vi "set poisition.vi"(4 "Mode":u16(ring) items=["Move to position", "Move to limit", "Redefine current position"], 5 "Instrument":T1={"325 Resource "="GPIB0::13::INSTR", "Input (0:A) 325"=0, "Heater Output (1:1) 325"=1, "340 Resource"="GPIB0::14::INSTR", "Input (0:A) 340"=0, "Loop (0: 1)"=0, "Input (0:B) 340"=1, "Loop (1: 1)"=0, "340 Status"=refnum, "Instrument Type"=enum."PPMS-Rotate", "quantum design"=refnum, "semaphore 325"=refnum, "TCP master instance"=refnum, "M24C Resource"="GPIB0::24::INSTR", "4G supply"="GPIB0::24::INSTR", "Temp Status 24C"=refnum, "Temp"=refnum, "9T信号"=refnum, "limit"={"Field limit"=0.0, "Field rate limit"=0.0, "Temp limit"=0.0, "Temp low limit"=0.0, "Temp rate limit "=0.0}, "4g supply status"=refnum, "vi路径"="", "in-plane"="", "out-plane"="", "in-plane signal"=FALSE, "out-plane signal"=FALSE, "in plane 信号"=refnum, "pzt volt"=refnum, "Aborting"=refnum, "数据文件"=refnum, "warning"=refnum, "750 visa"="", "750 rotate"="", "335 Status 2"=refnum, "335 Resource "="GPIB0::24::INSTR", "Input (0:A) 335"=0, "Input (0:B) 335"=1, "Heater Output (1:1) 335"=1, "semaphore 340"=refnum, "semaphore 335"=refnum, "325 Status"=refnum, "semaphore 750"=refnum, "750 field status"=refnum, "camg 振荡状态"=refnum, "列表框"=refnum, "编辑列表框？"=refnum, "camg Rate"=refnum, "行数"=refnum, "TM620"="TCPIP0::192.168.1.5::4266::SOCKET"} {"Loop (1: 1)" items=["1"=1, "2"=2]; "Loop (0: 1)" items=["1"=1, "2"=2]; "Input (0:B) 340" items=["A", "B", "C", "D"]; "Heater Output (1:1) 335" items=["1"=1, "2"=2]; "Input (0:B) 335" items=["A", "B"]; "Input (0:A) 335" items=["A", "B"]; "Heater Output (1:1) 325" items=["1"=1, "2"=2]; "Input (0:A) 325" items=["A", "B"]; "Input (0:A) 340" items=["1"=1, "2"=2]}, 6 "Slow down code\ndefault = 0":T5(ring), 7 "Position (deg)":dbl, 8 "error in (no error)":errorcluster, 9 "Instrument Ref In":refnum<k24>) -> (2 "error out":errorcluster, 3 "Instrument Ref Out":refnum<k24>)   [LabVIEW 2019, in "SubVI.lvlib"]
uses:
  SubVI.lvlib
  C:/Users/fuyang/Desktop/postdoctor/labview/labview-measure/lib/QDInstrument.dll
  lib/QDInstrument.dll
  ctl/Instrument.ctl
  <vilib>/NI/Modbus Library/API/Master/Modbus Master.lvclass
  ctl/335 state.ctl
  ctl/Instrument Type.ctl
  ctl/limit.ctl
  ctl/9T mag field stauts.ctl
  ctl/warning.ctl
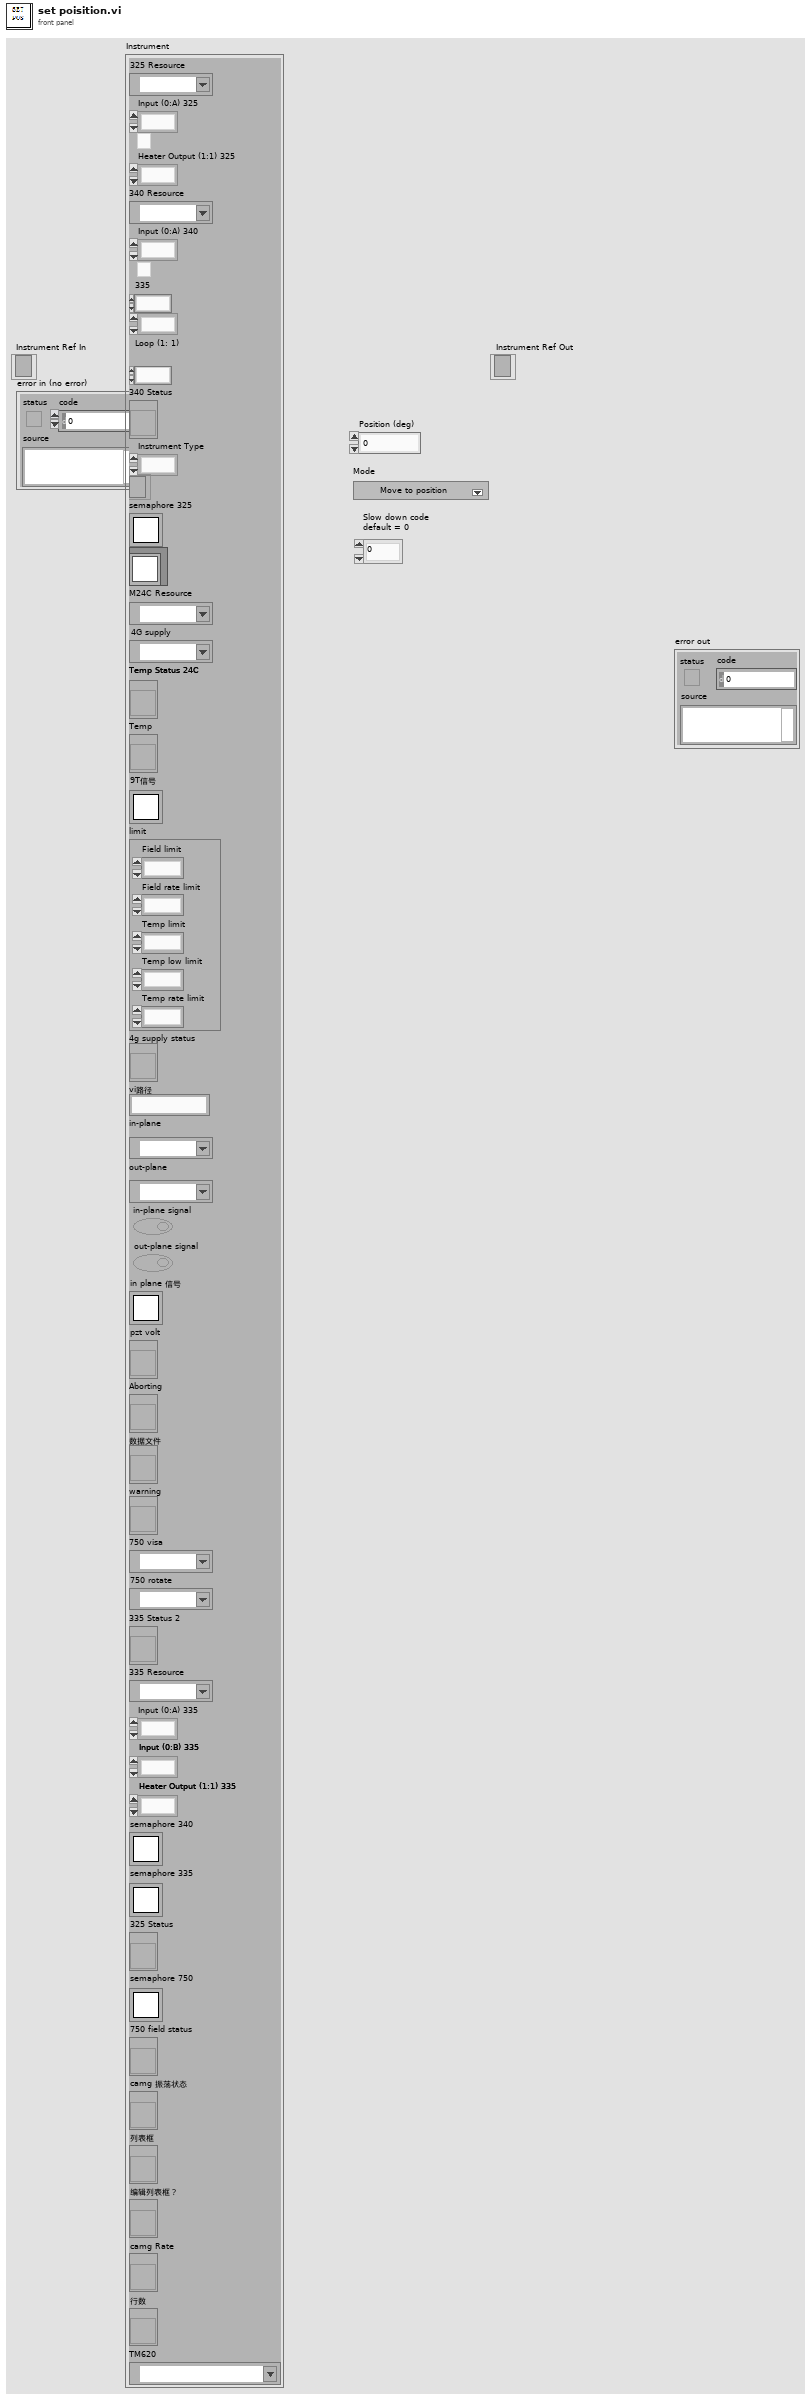
[diagram p1: front panel]
types:
  T1 = typedef "Instrument.ctl" = cluster{"325 Resource ":refnum<visa-resource-name>, "Input (0:A) 325":u16, "Heater Output (1:1) 325":u16, "340 Resource":refnum<visa-resource-name>, "Input (0:A) 340":u16, "Loop (0: 1)":u16, "Input (0:B) 340":u16, "Loop (1: 1)":u16, "340 Status":refnum<vi>, "Instrument Type":T2, "quantum design":refnum<k24>, "semaphore 325":T3, "TCP master instance":refnum<class "Modbus Master.lvclass">, "M24C Resource":refnum<visa-resource-name>, "4G supply":refnum<visa-resource-name>, "Temp Status 24C":refnum<vi>, "Temp":refnum<vi>, "9T信号":T3, "limit":T4, "4g supply status":refnum<vi>, "vi路径":string, "in-plane":refnum<visa-resource-name>, "out-plane":refnum<visa-resource-name>, "in-plane signal":bool, "out-plane signal":bool, "in plane 信号":T3, "pzt volt":refnum<vi>, "Aborting":refnum<vi>, "数据文件":refnum<vi>, "warning":refnum<vi>, "750 visa":refnum<visa-resource-name>, "750 rotate":refnum<visa-resource-name>, "335 Status 2":refnum<vi>, "335 Resource ":refnum<visa-resource-name>, "Input (0:A) 335":u16, "Input (0:B) 335":u16, "Heater Output (1:1) 335":u16, "semaphore 340":T3, "semaphore 335":T3, "325 Status":refnum<vi>, "semaphore 750":T3, "750 field status":refnum<vi>, "camg 振荡状态":refnum<vi>, "列表框":refnum<vi>, "编辑列表框？":refnum<vi>, "camg Rate":refnum<vi>, "行数":refnum<vi>, "TM620":refnum<visa-resource-name>}
  T2 = typedef "Instrument Type.ctl" = enum16{"PPMS", "VersaLab", "DynaCool", "SVSM", "PPMS-Rotate", "Lakeshore335", "lengtou2", "9T mag old", "9T cmag", "9T cmag DAC", "9T cmag rotate", "test"}
  T3 = typedef "Semaphore RefNum" = refnum<k1>
  T4 = typedef "limit.ctl" = cluster{"Field limit":dbl, "Field rate limit":dbl, "Temp limit":dbl, "Temp low limit":dbl, "Temp rate limit ":dbl}
  T5 = enum16{"0", "1", "2", "3", "4", "5", "6", "7", "8", "9", "10", "11", "12", "13", "14"}
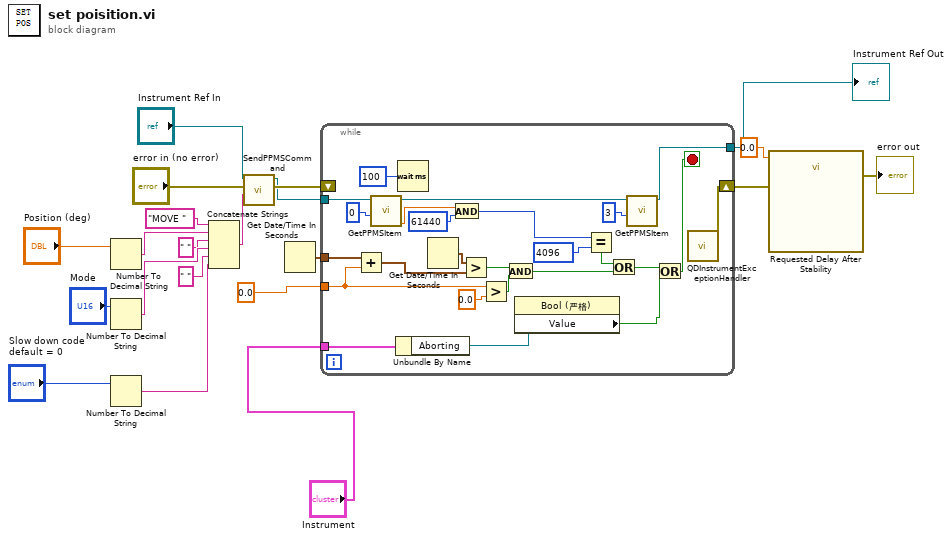
[diagram p0: block diagram]
diagram:
  n1 = Number To Decimal String(number="Position (deg)") -> (decimal integer string=w10:string)  [unwired: 1 in]
  n2 = Number To Decimal String(number="Mode") -> (decimal integer string=w13:string)  [unwired: 1 in]
  n3 = Number To Decimal String(number="Slow down code\ndefault = 0") -> (decimal integer string=w16:string)  [unwired: 1 in]
  n4 = Concatenate Strings("MOVE " ("string"), w10, " " ("string"), w13, " " ("string"), w16) -> (w17:string)
  n5 = call "SendPPMSCommand.vi"("PpmsCommand"=w17, "error in (no error)"="error in (no error)", "Instrument Ref In"="Instrument Ref In") -> ("error out"=w21:errorcluster, "Instrument Ref Out"=w20:refnum<k24>)  [unwired: 4 in, 3 out]
  n6 = Get Date/Time In Seconds() -> (seconds since 1Jan1904=w19:timestamp)
  n7 = while {
    shift-right: [w37] -> w18
    shift-left: w21 -> [_]
    tunnel: w19 -> [w45]
    tunnel: 0.0 ("Timeout") -> [w42]
    tunnel: w20 -> [w36]
    tunnel: [w27] -> w6
    tunnel: "Instrument" -> [w24]
    stop <- w25 stop-if-true
    n8 = Add(x=w45, y=w42) -> (x+y=w43:timestamp)
    n9 = call "GetPPMSItem.vi"("Channel"=0, "Instrument Ref In"=w36) -> ("Result"=w30:dbl, "Instrument Ref Out"=w28:refnum<k24>)  [unwired: 2 in, 2 out]
    n10 = Unbundle By Name(w24) -> ("Aborting"=w23:refnum<vi>)
    n11 = Wait (ms)(milliseconds to wait=u32 100) -> ()  [unwired: 1 out]
    n12 = Get Date/Time In Seconds() -> (seconds since 1Jan1904=w44:timestamp)
    n13 = And(x=w30, y=61440) -> (x .and. y?=w34:i32)
    n14 = Greater?(x=w44, y=w43) -> (0:w40:bool)
    n15 = Greater?(x=w42, y=0.0) -> (0:w39:bool)
    n16 = And(x=w40, y=w39) -> (x .and. y?=w38:bool)
    n17 = property class="Bool (严格)"(reference=w23) -> ("Value"=w22:bool)  [unwired: 1 in, 2 out]
    n18 = Equal?(x=w34, y=4096) -> (x = y?=w32:bool)
    n19 = Or(x=w32, y=w38) -> (x .or. y?=w26:bool)
    n20 = call "GetPPMSItem.vi"("Channel"=3, "Instrument Ref In"=w28) -> ("Instrument Ref Out"=w27:refnum<k24>)  [unwired: 2 in, 3 out]
    n21 = Or(x=w26, y=w22) -> (x .or. y?=w25:bool)
    n22 = call "QDInstrumentExceptionHandler.vi"() -> ("Error out"=w37:errorcluster)  [unwired: 1 in]
  }
  "Instrument Ref Out" <- w6
  n23 = call "Requested Delay After Stability"("error in (no error)"=w18, "Delay Time (s)"=0.0) -> ("error out"=→"error out":errorcluster)  [unwired: 9 in]
